vi "PixyGetCube.vi"(10 "AbortButtonPushed":bool, 11 "CubeGrabButtonPushed":bool) -> (3 "GotCube?":bool)   [LabVIEW 2017]
uses:
  <vilib>/Rock Robotics/SystemInterfaces/i2clib/i2c_bus.ctl
panel:
  in  "EndCondArea":i32=11000
  in  "CenterSetpoint":i32=80
  in  "AreaSetpoint":i32
  in  "MaxY":i32=130
  in  "KdX":dbl=0.07
  in  "MaxSpeed":dbl=0.3
  in  "KpX":dbl=0.1
  in  "KpY":dbl=0.0001
  in  "Pixy Address":u8=84 format="%x"
  # "320 x 200"
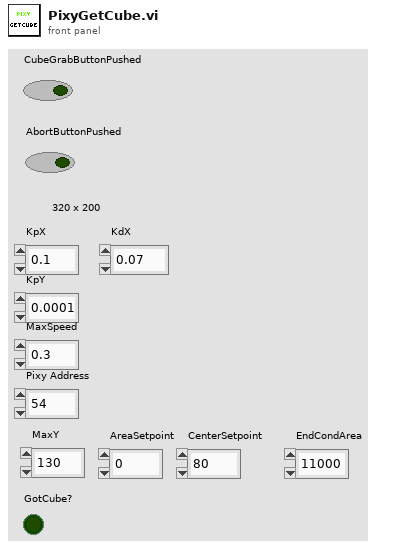
[diagram p1: front panel]
types:
  T1 = typedef "i2c_bus.ctl" = enum16{"I2C On-Board", "I2C MXP", "Invalid"}
  T2 = typedef "WPI_MotorControlDeviceRef.ctl" = cluster{"DeviceStatus":errorcluster, "Type":T3, "PWM":cluster{"PWM Channel":T4, "DeadBand":T5}, "CAN":cluster{"Device Number":u8, "SetOutput VI Ref":variant, "GetOutput VI Ref":variant, "Enable VI Ref":variant, "Disable VI Ref":variant, "Data":variant}, "Invert":bool, "DIO PWM":cluster{"PWM \"Enable\" Channel":T4, "DIOChannel":T6, "PWM Rate":dbl}}
  T3 = typedef "WPI_MotorControlType.ctl" = enum16{"PWM", "CAN", "DIO PWM"}
  T4 = typedef "FPGA_DIOPWMChannel.ctl" = enum8{"PWM 0", "PWM 1", "PWM 2", "PWM 3", "PWM 4", "PWM 5", "PWM 6", "PWM 7", "PWM 8", "PWM 9", "PWM MXP 0", "PWM MXP 1", "PWM MXP 2", "PWM MXP 3", "PWM MXP 4", "PWM MXP 5", "PWM MXP 6", "PWM MXP 7", "PWM MXP 8", "PWM MXP 9", "Invalid"}
  T5 = typedef "WPI_PWMDeadband.ctl" = cluster{"Name":string, "maxPositivePwm":i32, "minPositivePwm":i32, "centerPwm":i32, "maxNegativePwm":i32, "minNegativePwm":i32, "angularRange":u16}
  T6 = typedef "FPGA_DIOChannel.ctl" = enum8{"DIO 0", "DIO 1", "DIO 2", "DIO 3", "DIO 4", "DIO 5", "DIO 6", "DIO 7", "DIO 8", "DIO 9", "DIO MXP 0", "DIO MXP 1", "DIO MXP 2", "DIO MXP 3", "DIO MXP 4", "DIO MXP 5", "DIO MXP 6", "DIO MXP 7", "DIO MXP 8", "DIO MXP 9", "DIO MXP 10", "DIO MXP 11", "DIO MXP 12", "DIO MXP 13", "DIO MXP 14", "DIO MXP 15", "SPI Port CS1", "SPI Port CS2", "SPI Port CS3", "SPI Port MISO", "SPI Port MOSI", "Invalid"}
  T7 = typedef "WPI_I2CDevRef.ctl" = cluster{"DevStatus":errorcluster, "Device Address":u8, "Handle":i32, "I2C Bus":T1}
  T8 = cluster{"MotorControlDevRef":T2, "MotorControlDevRef":T2}
  T9 = cluster{"MotorControlDevRef":T2, "MotorControlDevRef":T2, "MotorControlDevRef":T2, "MotorControlDevRef":T2}
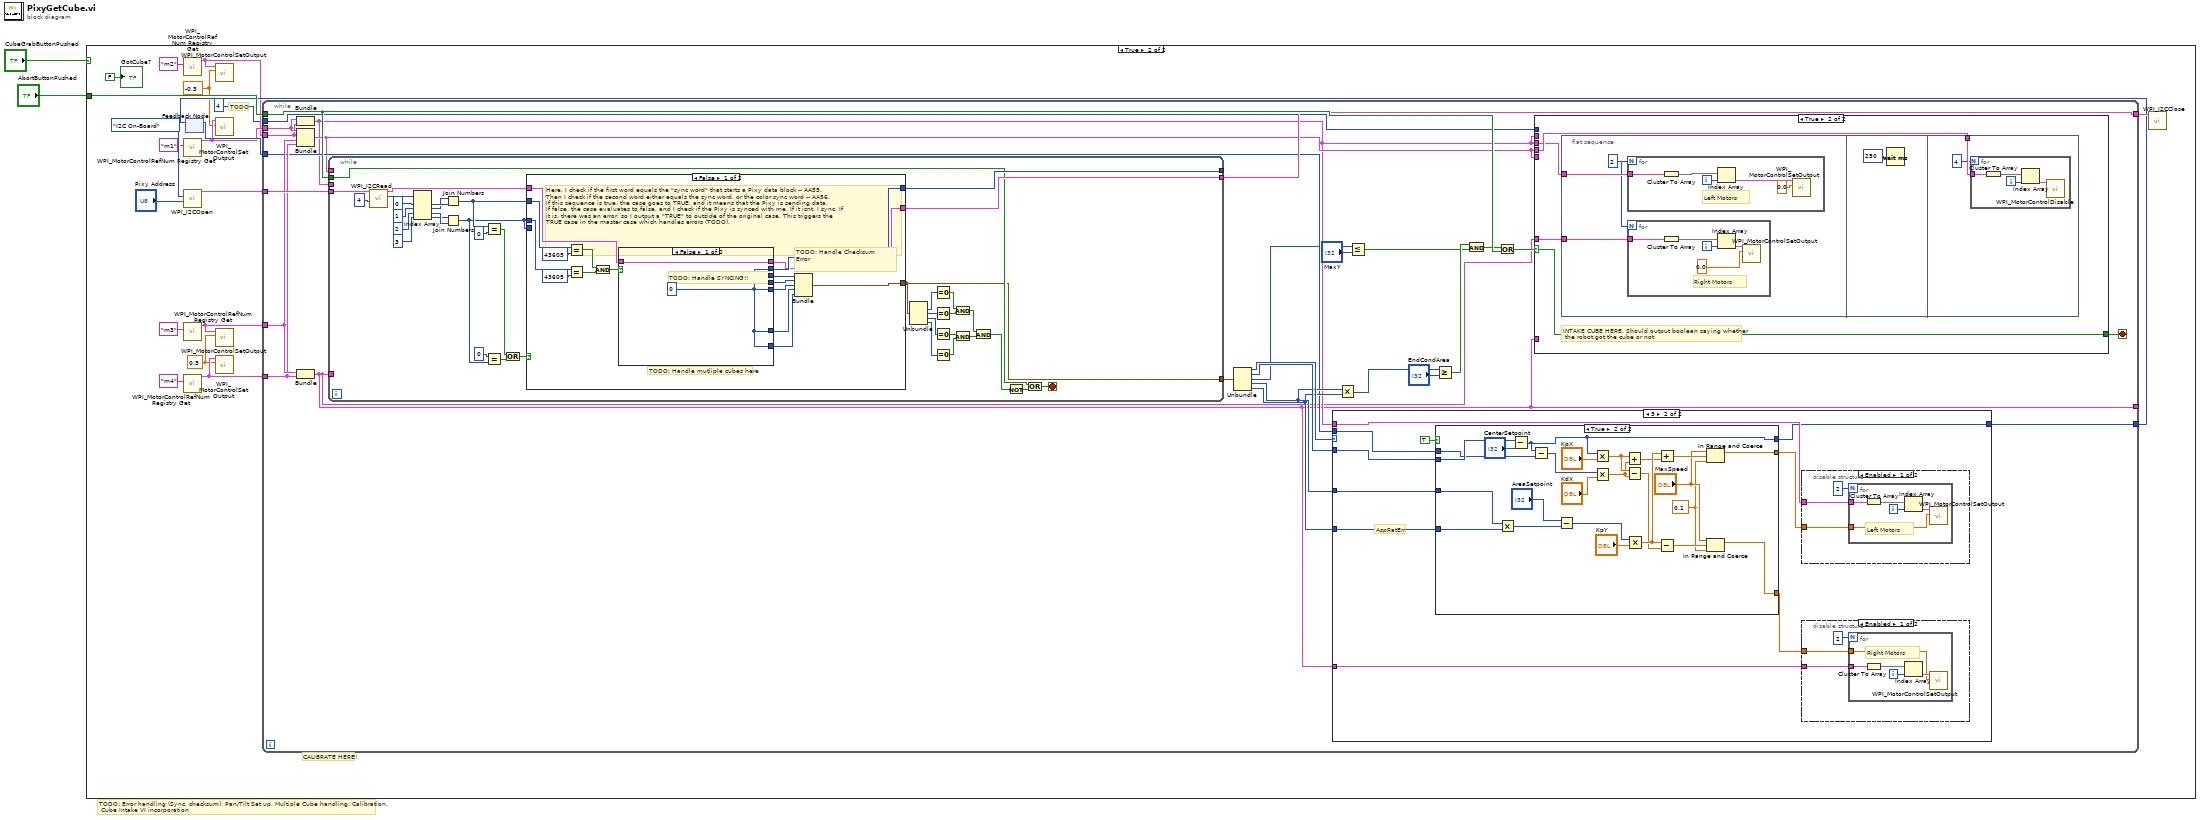
[diagram p0: block diagram]
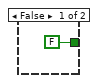
[diagram p3: hidden frame]
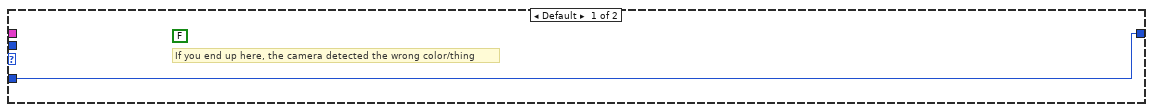
[diagram p4: hidden frame]
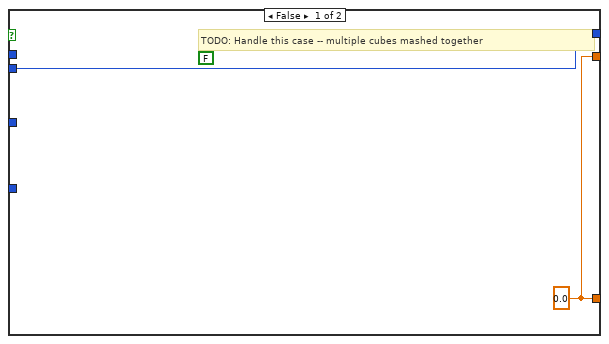
[diagram p7: hidden frame]
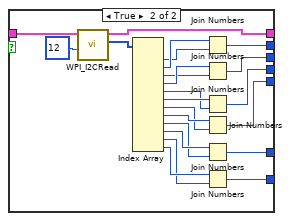
[diagram p8: hidden frame]
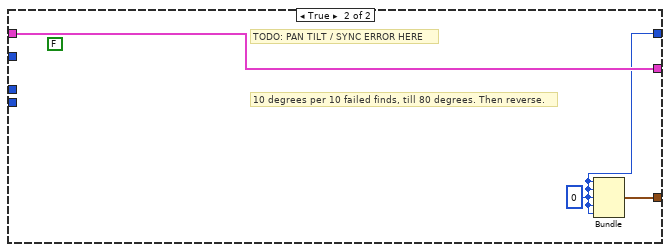
[diagram p9: hidden frame]
diagram:
  # "TODO: Error handling (Sync, checksum), Pan/Tilt Set up, Multiple Cube handling, Calibration,\n Cube Intake VI incorporation"
  n1 = case shown="True" "CubeGrabButtonPushed" {
    tunnel: "AbortButtonPushed" -> [_ w21]
    frame False {
    }
    frame True {
      w4 = -0.3 ("Output")
      w7 = 0.3 ("Output")
      # "TODO"
      # "CALIBRATE HERE!"
      n2 = call <vilib>:"WPI_MotorControlRefNum Registry Get.vi"("refnum name"="m2") -> ("MotorControlDevRef"=w5:T2)  [unwired: 9 in, 1 out]
      n3 = call <vilib>:"WPI_MotorControlRefNum Registry Get.vi"("refnum name"="m1") -> ("MotorControlDevRef"=w6:T2)  [unwired: 9 in, 1 out]
      n4 = call <vilib>:"WPI_I2COpen.vi"("Device Address"="Pixy Address", "I2C Bus"=i2c_bus."I2C On-Board") -> ("I2CDevRef"=w12:T7)  [unwired: 8 in, 1 out]
      n5 = call <vilib>:"WPI_MotorControlRefNum Registry Get.vi"("refnum name"="m3") -> ("MotorControlDevRef"=w9:T2)  [unwired: 9 in, 1 out]
      n6 = call <vilib>:"WPI_MotorControlRefNum Registry Get.vi"("refnum name"="m4") -> ("MotorControlDevRef"=w8:T2)  [unwired: 9 in, 1 out]
      n7 = feedback #1() -> (w11:i32)  [unwired: 1 in]
      n8 = call <vilib>:"WPI_MotorControlSetOutput.vi"("Output"=w4, "MotorControlDevRef"=w5) -> ()  [unwired: 7 in, 3 out]
      n9 = call <vilib>:"WPI_MotorControlSetOutput.vi"("Output"=w4, "MotorControlDevRef"=w6) -> ()  [unwired: 7 in, 3 out]
      n10 = call <vilib>:"WPI_MotorControlSetOutput.vi"("Output"=w7, "MotorControlDevRef"=w9) -> ()  [unwired: 7 in, 3 out]
      n11 = call <vilib>:"WPI_MotorControlSetOutput.vi"("Output"=w7, "MotorControlDevRef"=w8) -> ()  [unwired: 7 in, 3 out]
      n12 = while {
        tunnel: w21 -> [w48]
        tunnel: w5 -> [w39]
        tunnel: w6 -> [w40]
        tunnel: w8 -> [w37]
        tunnel: w9 -> [w38]
        tunnel: [w47] -> w18
        tunnel: w12 -> [w46]
        tunnel: [w24] -> _
        tunnel: w11 -> [w36]
        tunnel: [w35] -> w10
        tunnel: 4 -> [w27]
        stop <- w28 stop-if-true
        n13 = Bundle("MotorControlDevRef"=w40, "MotorControlDevRef"=w39) -> (w25:T8)  [unwired: 1 in]
        n14 = Bundle("MotorControlDevRef"=w40, "MotorControlDevRef"=w39, "MotorControlDevRef"=w38, "MotorControlDevRef"=w37) -> (w26:T9)  [unwired: 1 in]
        n15 = Bundle("MotorControlDevRef"=w38, "MotorControlDevRef"=w37) -> (w24:T8)  [unwired: 1 in]
        n16 = while {
          tunnel: w48 -> [w141]
          tunnel: w46 -> [w148]
          tunnel: [w143] -> _
          tunnel: [w142] -> w47
          tunnel: [w129] -> w43
          tunnel: w26 -> [_]
          tunnel: w25 -> [_]
          tunnel: w24 -> [_]
          stop <- w130 stop-if-true
          n17 = call <vilib>:"WPI_I2CRead.vi"("I2CBytesToRead"=u8 4, "I2CDevRef"=w148) -> ("Data Out"=w157:u8[], "I2CDevRef"=w146:T7)  [unwired: 7 in, 1 out]
          n18 = Index Array(array=w157, index #1=0 ("index"), index #2=1 ("index"), index #3=2 ("index"), index #4=3 ("index")) -> (element #1=w152:u8, element #2=w151:u8, element #3=w150:u8, element #4=w149:u8)
          n19 = Join Numbers(hi=w151, lo=w152) -> ((hi.lo)=w145:u16)
          n20 = Join Numbers(hi=w149, lo=w150) -> ((hi.lo)=w144:u16)
          n21 = Equal?(x=w145, y=u16 0) -> (x = y?=w160:bool)
          n22 = Equal?(x=u16 0, y=w144) -> (x = y?=w159:bool)
          n23 = Or(x=w160, y=w159) -> (x .or. y?=w147:bool)
          n24 = case shown="False" w147 {
            tunnel: w146 -> [w175 w205]
            tunnel: w145 -> [w174 _]
            tunnel: w144 -> [w173 _]
            tunnel: w144 -> [_ _]
            tunnel: [w172 w204] -> w143
            tunnel: [w169 w205] -> w142
            tunnel: [w163 w203] -> w129
            frame False {
              # "TODO: Handle Checksum \nError"
              # "TODO: Handle mutliple cubes here"
              # "Here, I check if the first word equals the \"sync word\" that starts a Pixy data block -- AA55. \nThen I check if the second word either equals the sync word, or the color sync word -- AA56.\nIf this sequence is true, the case goes to TRUE, and it means that the Pixy is sending data.\nIf false, the case evaluates to false, and I check if the Pixy is synced with me. If it isnt, I sync. If\nit is, there was an error, so I output a \"TRUE\" to outside of the original case. This triggers the \nTRUE case in the master case which handles errors (TODO)."
              n25 = Equal?(x=w174, y=u16 43605) -> (x = y?=w178:bool)
              n26 = Equal?(x=w173, y=u16 43605) -> (x = y?=w171:bool)
              n27 = And(x=w178, y=w171) -> (x .and. y?=w170:bool)
              n28 = case shown="False" w170 {
                tunnel: w175 -> [w179 w202]
                tunnel: [w180 w188] -> w164
                tunnel: [w180 w187] -> w165
                tunnel: [w180 w186] -> w166
                tunnel: [w180 w185] -> w167
                tunnel: [w180 w184] -> w168
                tunnel: [w180 w183] -> w172
                tunnel: [w179 w181] -> w169
                frame False {
                  w180 = 0
                  # "TODO: Handle SYNCING!!"
                }
                frame True {
                  n29 = call <vilib>:"WPI_I2CRead.vi"("I2CBytesToRead"=u8 12, "I2CDevRef"=w202) -> ("Data Out"=w182:u8[], "I2CDevRef"=w181:T7)  [unwired: 7 in, 1 out]
                  n30 = Index Array(array=w182) -> (element #1=w189:u8, element #2=w190:u8, element #3=w191:u8, element #4=w192:u8, element #5=w193:u8, element #6=w194:u8, element #7=w195:u8, element #8=w196:u8, element #9=w197:u8, element #10=w198:u8, element #11=w199:u8, element #12=w200:u8)  [unwired: 12 in]
                  n31 = Join Numbers(hi=w190, lo=w189) -> ((hi.lo)=w183:u16)
                  n32 = Join Numbers(hi=w192, lo=w191) -> ((hi.lo)=w184:u16)
                  n33 = Join Numbers(hi=w194, lo=w193) -> ((hi.lo)=w185:u16)
                  n34 = Join Numbers(hi=w196, lo=w195) -> ((hi.lo)=w186:u16)
                  n35 = Join Numbers(hi=w198, lo=w197) -> ((hi.lo)=w187:u16)
                  n36 = Join Numbers(hi=w200, lo=w199) -> ((hi.lo)=w188:u16)
                }
              }
              n37 = Bundle(w168, w167, w166, w165, w164) -> (w163:cluster{i32, i32, i32, i32, i32})  [unwired: 1 in]
            }
            frame True {
              (unwired) FALSE
              w204 = 0
              # "10 degrees per 10 failed finds, till 80 degrees. Then reverse."
              # "TODO: PAN TILT / SYNC ERROR HERE"
              n38 = Bundle(w204, w204, w204, w204, w204) -> (w203:cluster{i32, i32, i32, i32, i32})  [unwired: 1 in]
            }
          }
          n39 = Unbundle(w129) -> (w140:i32, w139:i32, w138:i32, w137:i32)  [unwired: 1 out]
          n40 = Equal To 0?(x=w140) -> (x = 0?=w128:bool)
          n41 = Equal To 0?(x=w139) -> (x = 0?=w136:bool)
          n42 = Equal To 0?(x=w138) -> (x = 0?=w135:bool)
          n43 = Equal To 0?(x=w137) -> (x = 0?=w134:bool)
          n44 = And(x=w128, y=w136) -> (x .and. y?=w132:bool)
          n45 = And(x=w135, y=w134) -> (x .and. y?=w131:bool)
          n46 = And(x=w132, y=w131) -> (x .and. y?=w127:bool)
          n47 = Not(x=w127) -> (.not. x?=w133:bool)
          n48 = Or(x=w141, y=w133) -> (x .or. y?=w130:bool)
        }
        n49 = Unbundle(w43) -> (w45:i32, w44:i32, w30:i32, w42:i32, w41:i32)
        n50 = case shown="3" w45 {
          tunnel: w24 -> [_ w84]
          tunnel: w25 -> [_ w83]
          tunnel: w44 -> [w74 w82]
          tunnel: w42 -> [_ w78]
          tunnel: w41 -> [_ w77]
          tunnel: [w74 w76] -> w35
          tunnel: w36 -> [_ w75]
          frame Default {
            (unwired) FALSE
            # "If you end up here, the camera detected the wrong color/thing"
          }
          frame 3 {
            # "AspRatErr"
            n51 = case shown="True" TRUE {
              tunnel: w82 -> [w101 w118]
              tunnel: [w102 w119] -> w80
              tunnel: [w102 w120] -> w81
              tunnel: w78 -> [_ w126]
              tunnel: w77 -> [_ w125]
              tunnel: [w101 w111] -> w76
              tunnel: w75 -> [_ w110]
              frame False {
                (unwired) FALSE
                w102 = 0.0
                # "TODO: Handle this case -- multiple cubes mashed together"
              }
              frame True {
                w105 = 0.1 ("lower limit")
                n52 = Multiply(x=w126, y=w125) -> (x*y=w116:i32)
                n53 = Subtract(x=w118, y="CenterSetpoint") -> (x-y=w111:i32)
                n54 = Subtract(x=w111, y=w110) -> (x-y=w112:i32)
                n55 = Subtract(x="AreaSetpoint", y=w116) -> (x-y=w115:i32)
                n56 = Multiply(x=w111, y="KpX") -> (x*y=w109:dbl)
                n57 = Multiply(x=w112, y="KdX") -> (x*y=w108:dbl)
                n58 = Add(x=w109, y=w108) -> (x+y=w113:dbl)
                n59 = Subtract(x=w109, y=w108) -> (x-y=w107:dbl)
                n60 = Multiply(x=w115, y="KpY") -> (x*y=w117:dbl)
                n61 = Add(x=w117, y=w113) -> (x+y=w122:dbl)
                n62 = Subtract(x=w117, y=w107) -> (x-y=w121:dbl)
                n63 = In Range and Coerce(upper limit="MaxSpeed", x=w122, lower limit=w105) -> (coerced(x)=w119:dbl)  [unwired: 1 out]
                n64 = In Range and Coerce(upper limit="MaxSpeed", x=w121, lower limit=w105) -> (coerced(x)=w120:dbl)  [unwired: 1 out]
              }
            }
            n65 = disable-structure shown="Enabled" {
              disable-tunnel: w83 -> [w94 _]
              disable-tunnel: w80 -> [w93 _]
              frame Enabled {
                n66 = for {
                  N: 2 -> [_]
                  tunnel: w94 -> [w96]
                  tunnel: w93 -> [w97]
                  i -> [w98]
                  # "Left Motors"
                  n67 = Cluster To Array(cluster=w96) -> (array=w100:T2[])
                  n68 = Index Array(array=w100, index=w98) -> (element=w99:T2)
                  n69 = call <vilib>:"WPI_MotorControlSetOutput.vi"("Output"=w97, "MotorControlDevRef"=w99) -> ()  [unwired: 7 in, 3 out]
                }
              }
              frame Disabled {
              }
            }
            n70 = disable-structure shown="Enabled" {
              disable-tunnel: w84 -> [w86 _]
              disable-tunnel: w81 -> [w85 _]
              frame Enabled {
                n71 = for {
                  N: 2 -> [_]
                  tunnel: w86 -> [w88]
                  tunnel: w85 -> [w89]
                  i -> [w91]
                  # "Right Motors"
                  n72 = Cluster To Array(cluster=w88) -> (array=w92:T2[])
                  n73 = Index Array(array=w92, index=w91) -> (element=w90:T2)
                  n74 = call <vilib>:"WPI_MotorControlSetOutput.vi"("Output"=w89, "MotorControlDevRef"=w90) -> ()  [unwired: 7 in, 3 out]
                }
              }
              frame Disabled {
              }
            }
          }
        }
        n75 = Multiply(x=w42, y=w41) -> (x*y=w31:i32)
        n76 = Less Or Equal?(x=w30, y="MaxY") -> (x <= y?=w32:bool)
        n77 = Greater Or Equal?(x=w31, y="EndCondArea") -> (x >= y?=w34:bool)
        n78 = And(x=w34, y=w32) -> (x .and. y?=w33:bool)
        n79 = Or(x=w33, y=w48) -> (x .or. y?=w29:bool)
        n80 = case shown="True" w29 {
          selector: w29 -> [_ w53]
          tunnel: w27 -> [_ _]
          tunnel: w26 -> [_ _]
          tunnel: [FALSE w53] -> w28
          tunnel: w25 -> [_ _]
          tunnel: w24 -> [_ _]
          tunnel: w26 -> [_ w52]
          tunnel: w25 -> [_ w51]
          tunnel: w24 -> [_ w50]
          frame False {
          }
          frame True {
            # "INTAKE CUBE HERE. Should output boolean saying whether\n the robot got the cube or not"
            n81 = flat-sequence {
              tunnel: w51 -> [w56]
              tunnel: w50 -> [w55]
              tunnel: w52 -> [w69]
              frame #0 {
                w54 = 2
                n82 = for {
                  N: w54 -> [_]
                  tunnel: w56 -> [w63]
                  i -> [w64]
                  # "Left Motors"
                  n83 = Cluster To Array(cluster=w63) -> (array=w66:T2[])
                  n84 = Index Array(array=w66, index=w64) -> (element=w65:T2)
                  n85 = call <vilib>:"WPI_MotorControlSetOutput.vi"("Output"=0.0, "MotorControlDevRef"=w65) -> ()  [unwired: 7 in, 3 out]
                }
                n86 = for {
                  N: w54 -> [_]
                  tunnel: w55 -> [w58]
                  i -> [w60]
                  # "Right Motors"
                  n87 = Cluster To Array(cluster=w58) -> (array=w61:T2[])
                  n88 = Index Array(array=w61, index=w60) -> (element=w59:T2)
                  n89 = call <vilib>:"WPI_MotorControlSetOutput.vi"("Output"=0.0, "MotorControlDevRef"=w59) -> ()  [unwired: 7 in, 3 out]
                }
              }
              frame #1 {
                n90 = Wait (ms)(milliseconds to wait=u32 250) -> ()  [unwired: 1 out]
              }
              frame #2 {
                n91 = for {
                  N: 4 -> [_]
                  tunnel: w69 -> [w71]
                  i -> [w73]
                  n92 = Cluster To Array(cluster=w71) -> (array=w72:T2[])
                  n93 = Index Array(array=w72, index=w73) -> (element=w70:T2)
                  n94 = call <vilib>:"WPI_MotorControlDisable.vi"("MotorControlDevRef"=w70) -> ()  [unwired: 9 in, 2 out]
                }
              }
            }
          }
        }
      }
      n95 = feedback-in #1(w10) -> ()
      n96 = call <vilib>:"WPI_I2CClose.vi"("I2CDevRef"=w18) -> ()  [unwired: 10 in, 1 out]
      "GotCube?" <- FALSE ("GotCube?")
    }
  }
